vi "BuildCaseTagName.vi"(9 "Case Name":string, 10 "Parent Tag":string) -> (2 "Tag Name":string)   [LabVIEW 2019, in "ResultTree.lvclass"]
doc: "Returns the tag name for a test case. If no parent tag is specified (\"\"), the tag name is the same as the case name with prefix \"CASE_\". If a parent tag is specified, however, the tag name is the same as the parent tag followed by a \"/\" and the name of the case.\n\n<B>Examples</B>:\nparent: \"\"\ncase: \"My case\nresult: \"SUITE_My case\"\n\nparent: \"SUITE_My case\"\ncase: \"Another case\"\nresult: \"SUITE_My case/Another case\""
uses:
  ResultTree.lvclass
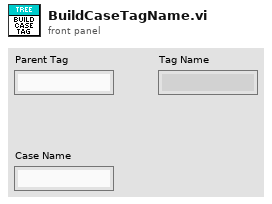
[diagram p1: front panel]
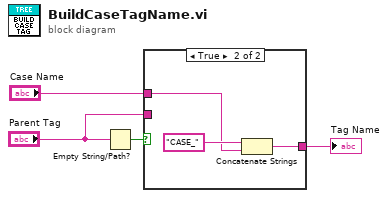
[diagram p0: block diagram]
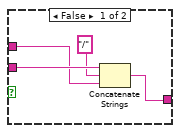
[diagram p2: hidden frame]
diagram:
  n1 = Empty String/Path?(string/path="Parent Tag") -> (empty?=w4:bool)
  n2 = case shown="True" w4 {
    tunnel: [w5 w10] -> w1
    tunnel: "Case Name" -> [w6 w9]
    tunnel: "Parent Tag" -> [w8 _]
    frame False {
      n3 = Concatenate Strings(w8, "/" ("string"), w6) -> (w5:string)
    }
    frame True {
      n4 = Concatenate Strings("CASE_", w9) -> (w10:string)
    }
  }
  "Tag Name" <- w1
